vi "Arduino Initialize Filter Wheel Table File.vi"   [LabVIEW 2021]
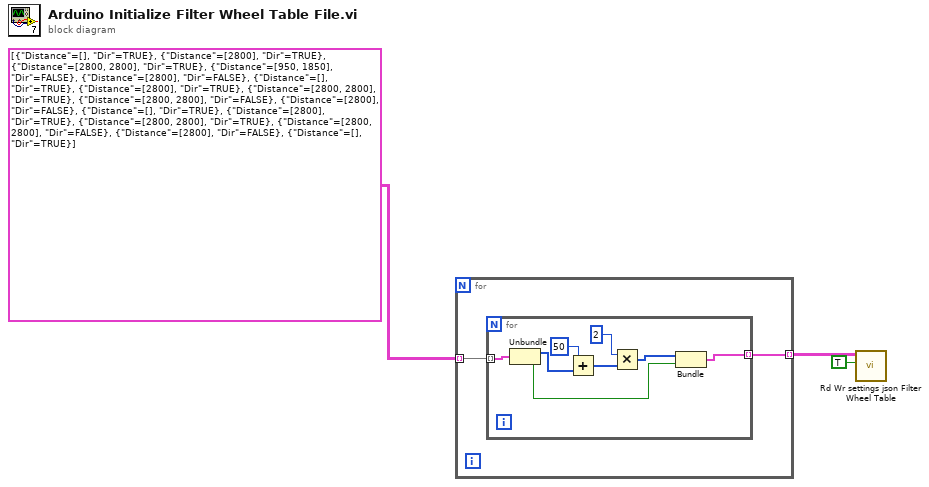
[diagram p0: block diagram]
diagram:
  n1 = for {
    tunnel: cluster{"Distance":i32[], "Dir":bool}[][] [[{"Distance"=[], "Dir"=TRUE}, {"Distance"=[2800], "Dir"=TRUE}, {"Distance"=[2800, 2800], "Dir"=TRUE}, {"Distance"=[950, 1850], "Dir"=FALSE}], [{"Distance"=[2800], "Dir"=FALSE}, {"Distance"=[], "Dir"=TRUE}, {"Distance"=[2800], "Dir"=TRUE}, {"Distance"=[2800, 2800], "Dir"=TRUE}], [{"Distance"=[2800, 2800], "Dir"=FALSE}, {"Distance"=[2800], "Dir"=FALSE}, {"Distance"=[], "Dir"=TRUE}, {"Distance"=[2800], "Dir"=TRUE}], [{"Distance"=[2800, 2800], "Dir"=TRUE}, {"Distance"=[2800, 2800], "Dir"=FALSE}, {"Distance"=[2800], "Dir"=FALSE}, {"Distance"=[], "Dir"=TRUE}]] -> [w5] mode=indexing
    tunnel: [w4] -> w2 mode=indexing
    n2 = for {
      tunnel: w5 -> [w13] mode=indexing
      tunnel: [w6] -> w4 mode=indexing
      n3 = Unbundle(w13) -> ("Distance"=w10:i32[], "Dir"=w7:bool)
      n4 = Add(x=50, y=w10) -> (x+y=w9:i32[])
      n5 = Multiply(x=2, y=w9) -> (x*y=w8:i32[])
      n6 = Bundle(w8, "Dir"=w7) -> (w6:cluster{i32[], "Dir":bool})  [unwired: 1 in]
    }
  }
  n7 = call "Rd Wr settings json Filter Wheel Table.vi"("Write? (F:Read)"=TRUE, "Filter Wheel Table"=w2) -> ()  [unwired: 8 in, 2 out]
